vi "Main Test.vi"(8 "error in (no error)":errorcluster) -> (0 "error out":errorcluster)   [LabVIEW 2020]
uses:
  <vilib>/addons/_JKI Toolkits/Caraya/classes/Test/Test.lvclass
  <vilib>/addons/_JKI Toolkits/Caraya/classes/Assert/Assert.lvclass
  <vilib>/addons/_JKI Toolkits/Caraya/classes/Assert/Assert Error.vi
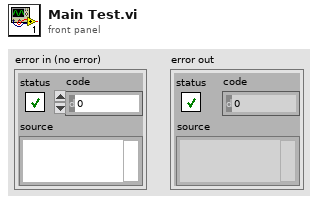
[diagram p1: front panel]
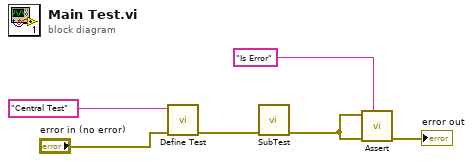
[diagram p0: block diagram]
diagram:
  n1 = call <vilib>:"Define Test.vi"("error in (no error)"="error in (no error)", "Label (VI Title)"="Central Test") -> ("error out"=w4:errorcluster)  [unwired: 8 in, 1 out]
  n2 = call "SubTest.vi"("error in (no error)"=w4) -> ("error out"=w3:errorcluster)  [unwired: 10 in]
  n3 = call-poly <vilib>:"Assert.vi"("Label"="Is Error", "error in (no error)"=w3, "Error?"=w3) -> ("error out"=→"error out":errorcluster)  [unwired: 7 in, 1 out]
